vi "TimedLauncher.vi"(4 "Scan Period":dbl format="%.2f", 5 "Previous Scan Value":dbl format="%.2f", 6 "Present scan array":dbl[](array[numeric]) format="%.2f", 7 "Value to Output":dbl format="%.2f", 8 "Ch Description":T1={"Ch Name"="", "Type"="Run VI Named:", "Function"=enum."Analogue Input", "Ch State"=enum."On", "Calibration type"="", "A"=0.0, "B"=0.0, "C"=0.0, "D"=0.0, "Comments"="TimedLauncher.vi", "Address"={"Main"=0, "Ch."=0, "Sub"=0, "Port Name"=""}, "String"="", "Duty"=0} {"Duty" format="%016b"; "D" format="%#_5g"; "C" format="%#_5g"; "B" format="%#_5g"; "A" format="%#_5g"}, 9 "Ch names":string[](array[string])) -> (0 "Scan comment":string, 1 "Output":dbl format="%.3f", 3 "HelpText":string="Add helpful help text here!")   [LabVIEW 2022 SP3]
uses:
  ADAM Client/Sub VIs/ADAM Controls/Ch_description_ADAM.ctl
  ADAM Client/Sub VIs/ADAM Controls/Module_type_ADAM.ctl
  ADAM Client/Sub VIs/ADAM Controls/Function_ADAM.ctl
  ADAM Client/Sub VIs/ADAM Controls/Channel_State.ctl
  ADAM Client/Sub VIs/ADAM Controls/Calib_type_ADAM.ctl
  ADAM Client/Sub VIs/ADAM Controls/Address.ctl
panel:
  out "DoItNow":bool
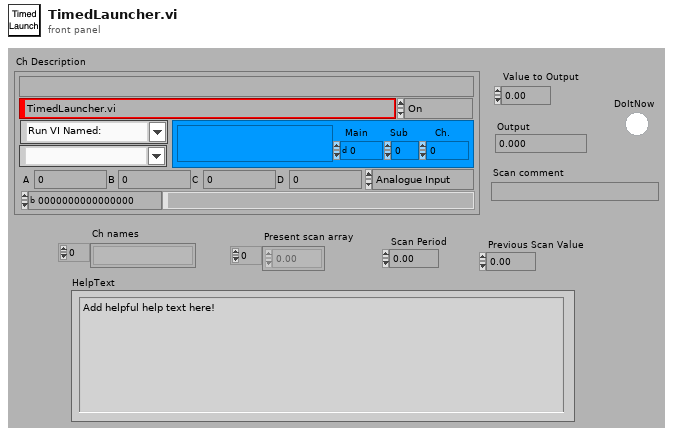
[diagram p1: front panel]
types:
  T1 = typedef "Ch_description_ADAM.ctl" = cluster{"Ch Name":string, "Type":T2, "Function":T3, "Ch State":T4, "Calibration type":T5, "A":dbl, "B":dbl, "C":dbl, "D":dbl, "Comments":string, "Address":T6, "String":string, "Duty":u16}
  T2 = typedef "Module_type_ADAM.ctl" = string
  T3 = typedef "Function_ADAM.ctl" = enum16{"Analogue Input", "Digital Input", "Event counter", "Event rate", "Analogue Output", "Digital Output", "Relay Output"}
  T4 = typedef "Channel_State.ctl" = enum16{"On", "Off", "Always On", "Always Off"}
  T5 = typedef "Calib_type_ADAM.ctl" = string
  T6 = typedef "Address.ctl" = cluster{"Main":i32, "Ch.":i32, "Sub":i32, "Port Name":string}
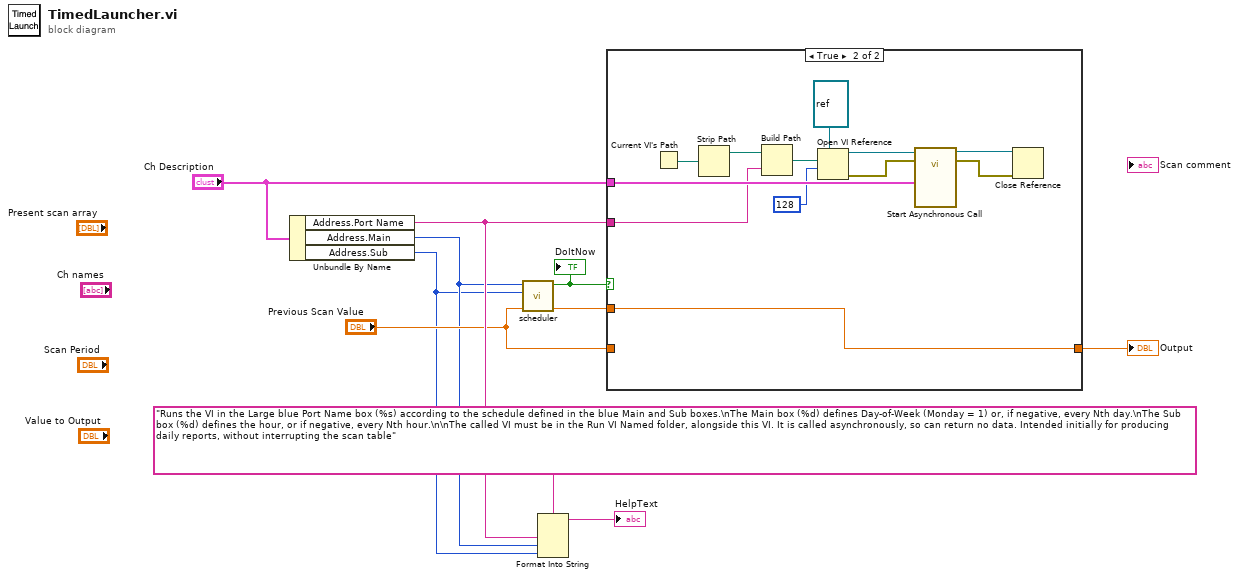
[diagram p0: block diagram]
diagram:
  n1 = Unbundle By Name("Ch Description") -> ("Address.Port Name"=w7:string, "Address.Main"=w2:i32, "Address.Sub"=w1:i32)
  n2 = call "scheduler.vi"("timestampLastFired"="Previous Scan Value", "Hour"=w1, "Day"=w2) -> ("timestampNow"=w3:dbl, "DoItNow"=w5:bool)  [unwired: 7 in]
  "DoItNow" <- w5
  n3 = Format Into String(format string="Runs the VI in the Large blue Port Name box (%s) according to the schedule defined in the blue Main and Sub boxes.\nThe Main box (%d) defines Day-of-Week (Monday = 1) or, if negative, every Nth day.\nThe Sub box (%d) defines the hour, or if negative, every Nth hour.\n\nThe called VI must be in the Run VI Named folder, alongside this VI. It is called asynchronously, so can return no data. Intended initially for producing daily reports, without interrupting the scan table", w7, w2, w1) -> (resulting string=→"HelpText":string)  [unwired: 2 in, 1 out]
  n4 = case shown="True" w5 {
    tunnel: "Ch Description" -> [_ w17]
    tunnel: w7 -> [_ w14]
    tunnel: w3 -> [_ w13]
    tunnel: [w11 w13] -> w9
    tunnel: "Previous Scan Value" -> [w11 _]
    frame False {
    }
    frame True {
      n5 = Current VI's Path() -> (path=w23:path)
      n6 = Strip Path(path=w23) -> (stripped path=w22:path)  [unwired: 1 out]
      n7 = Build Path(base path=w22, name or relative path=w14) -> (appended path=w21:path)
      n8 = Open VI Reference(type specifier VI Refnum (for type only)=refnum<vi> refnum, vi path=w21, options=128) -> (vi reference=w20:refnum<vi>, error out=w19:errorcluster)  [unwired: 3 in]
      n9 = call-by-ref "Start Asynchronous Call"(reference=w20, error in=w19, "Ch Description"=w17) -> (reference out=w16:refnum<vi>, error out=w15:errorcluster)  [unwired: 6 in, 3 out]
      n10 = Close Reference(reference=w16, error in (no error)=w15) -> ()  [unwired: 1 out]
    }
  }
  "Output" <- w9
